vi "AIP State Parser.vi"(9 "String":string) -> (3 "AIP States":T1)   [LabVIEW 2015, in "AIP Instrument.lvlib" / "AIP Instrument.lvclass"]
uses:
  AIP Instrument.lvclass
  Libraries/RDS Instruments/AIP/AIP States.ctl
  Libraries/RDS Instruments/RDS Instrument Library.lvlib
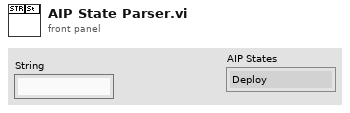
[diagram p1: front panel]
types:
  T1 = typedef "RDS Instrument Library.lvlib/AIP States.ctl" = enum16{"Deploy", "Deploying", "Deployed", "Stow", "Stowing", "Stowed", "Fault", "brakeOnStow", "breakOnDeploy", "Stopped", "Stopping"}
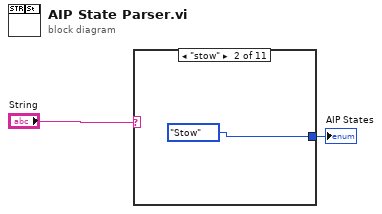
[diagram p0: block diagram]
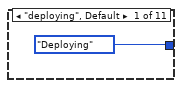
[diagram p2: hidden frame]
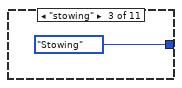
[diagram p3: hidden frame]
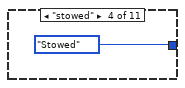
[diagram p4: hidden frame]
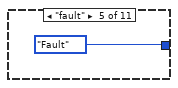
[diagram p5: hidden frame]
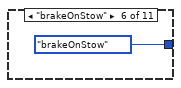
[diagram p6: hidden frame]
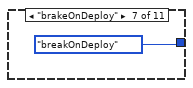
[diagram p7: hidden frame]
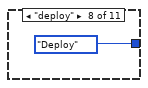
[diagram p8: hidden frame]
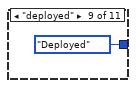
[diagram p9: hidden frame]
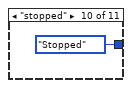
[diagram p10: hidden frame]
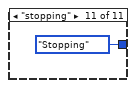
[diagram p11: hidden frame]
diagram:
  n1 = case shown="\"stow\"" "String" {
    tunnel: [AIP_States."Deploying" ("AIP States") AIP_States."Stow" ("AIP States") AIP_States."Stowing" ("AIP States") AIP_States."Stowed" ("AIP States") AIP_States."Fault" ("AIP States") AIP_States."brakeOnStow" ("AIP States") AIP_States."breakOnDeploy" ("AIP States") AIP_States."Deploy" ("AIP States") AIP_States."Deployed" ("AIP States") AIP_States."Stopped" ("AIP States") AIP_States."Stopping" ("AIP States")] -> w1
    frame "deploying", Default {
    }
    frame "stow" {
    }
    frame "stowing" {
    }
    frame "stowed" {
    }
    frame "fault" {
    }
    frame "brakeOnStow" {
    }
    frame "brakeOnDeploy" {
    }
    frame "deploy" {
    }
    frame "deployed" {
    }
    frame "stopped" {
    }
    frame "stopping" {
    }
  }
  "AIP States" <- w1
